vi "Configuration Dialog Box.vi"(8 "error in (no error)":errorcluster, 11 "Configuration Settings In":T1={"Signal type"=enum."Sine Wave", "Amplitude"=1.0, "Offset"=0.0, "Amplitude 2"=1.0, "Frequency"=10.0} {"Frequency" format="%0.2p"; "Amplitude 2" format="%.2p"; "Offset" format="%0.2p"; "Amplitude" format="%0.2p"}) -> (0 "error out":errorcluster, 3 "Configuration Settings Out":T1={"Signal type"=enum."Sine Wave", "Amplitude"=1.0, "Offset"=0.0, "Amplitude 2"=1.0, "Frequency"=10.0} {"Frequency" format="%0.2p"; "Amplitude 2" format="%.2p"; "Offset" format="%0.2p"; "Amplitude" format="%0.2p"})   [LabVIEW 2018]
uses:
  controls/Configuration Settings.ctl
panel:
  in  "Frequency":dbl=10.0 format="%0.2p"
  in  "Noise Amplitude":dbl=1.0 format="%.2p"
  in  "Offset":dbl format="%0.2p"
  in  "Amplitude":dbl=1.0 format="%0.2p"
  in  "Signal type":u16(ring) items=["Sine Wave", "Triangle Wave", "Square Wave", "Sawtooth Wave"]
  in  "Cancel":bool
  in  "Ok Button":bool
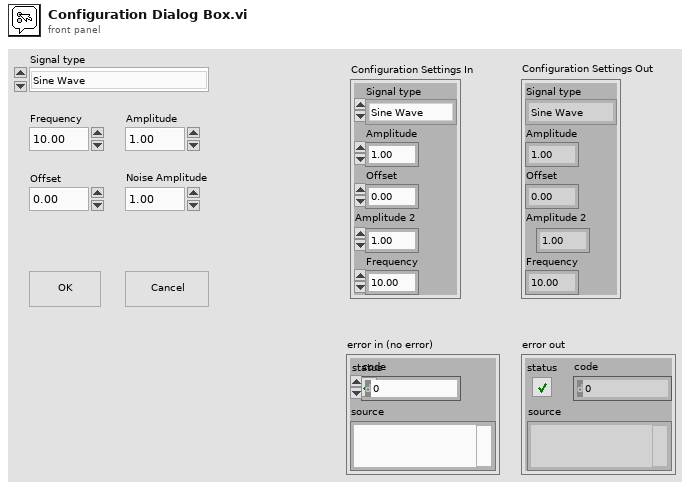
[diagram p1: front panel]
types:
  T1 = typedef "Configuration Settings.ctl" = cluster{"Signal type":enum16{"Sine Wave", "Triangle Wave", "Square Wave", "Sawtooth Wave"}, "Amplitude":dbl, "Offset":dbl, "Amplitude 2":dbl, "Frequency":dbl}
  T2 = enum16{"Sine Wave", "Triangle Wave", "Square Wave", "Sawtooth Wave"}
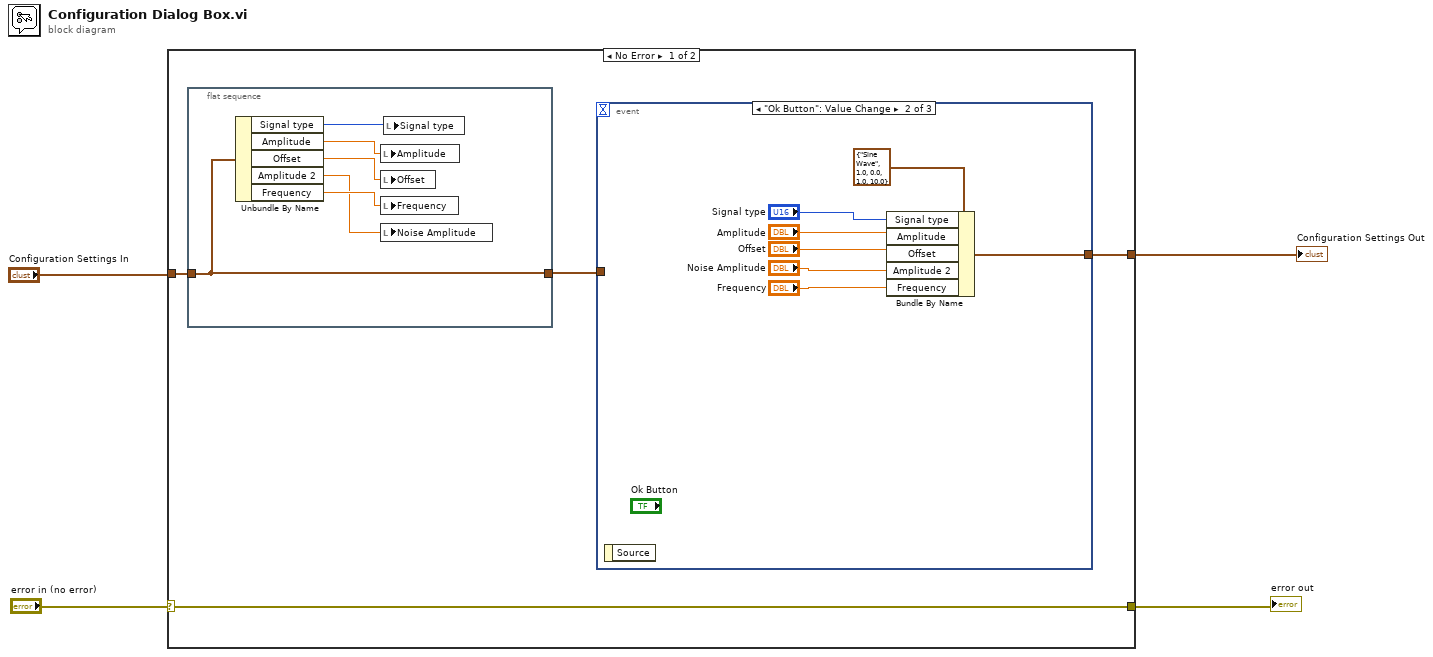
[diagram p0: block diagram]
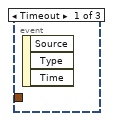
[diagram p2: hidden frame]
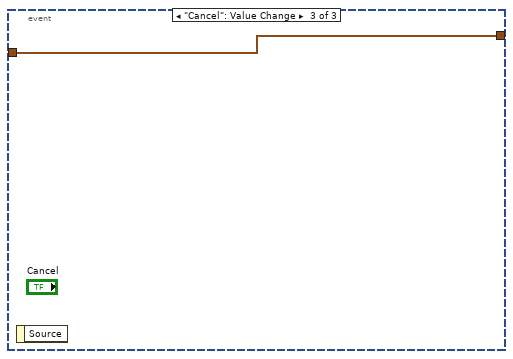
[diagram p3: hidden frame]
diagram:
  n1 = case shown="No Error" "error in (no error)" {
    selector: "error in (no error)" -> [w7 w22]
    tunnel: "Configuration Settings In" -> [w5 _]
    tunnel: [w7 w22] -> w2
    tunnel: [w6 _] -> w1
    frame No Error {
      n2 = flat-sequence {
        tunnel: w5 -> [w8]
        tunnel: [w8] -> _
        frame #0 {
          n3 = Unbundle By Name(w8) -> ("Signal type"=w11:T2, "Amplitude"=w13:dbl, "Offset"=w12:dbl, "Amplitude 2"=w9:dbl, "Frequency"=w10:dbl)
          n4 = local write "Amplitude"(w13) -> ()
          n5 = local write "Offset"(w12) -> ()
          n6 = local write "Frequency"(w10) -> ()
          n7 = local write "Noise Amplitude"(w9) -> ()
          n8 = local write "Signal type"(w11) -> ()
        }
      }
      n9 = event shown="[1] \"Ok Button\": Value Change" {
        selector: _ -> [_ _ _]
        dyn-events: _ -> [_ _ _]
        timeout: _ -> [_ _ _]
        tunnel: [_ w18 w21] -> w6
        tunnel: w5 -> [_ _ w21]
        event Timeout {
          n10 = event-data() -> ()  [unwired: 1 in, 3 out]
        }
        event "Ok Button": Value Change {
          n11 = event-data() -> ()  [unwired: 1 in, 1 out]
          n12 = Bundle By Name(cluster=T1 {"Signal type"=enum."Sine Wave", "Amplitude"=1.0, "Offset"=0.0, "Amplitude 2"=1.0, "Frequency"=10.0} ("Configuration Settings Out"), "Signal type"="Signal type", "Amplitude"="Amplitude", "Offset"="Offset", "Amplitude 2"="Noise Amplitude", "Frequency"="Frequency") -> (w18:T1)
        }
        event "Cancel": Value Change {
          n13 = event-data() -> ()  [unwired: 1 in, 1 out]
        }
      }
    }
    frame Error {
    }
  }
  "Configuration Settings Out" <- w1
  "error out" <- w2
